vi "NIIE_Classes Initialization.vi"(7 "LabVIEW Icon":string, 8 "Error":errorcluster {"code" min=0 max=0}, 10 "User Events":T8, 11 "Ref Cluster":T3) -> (0 "Error Out":errorcluster {"code" min=0 max=0}, 3 "Data Out":T1={"Class"={"Ants"=refnum, "Layer"=refnum, "Templates"=refnum, "Icon"=refnum, "Glyph"=refnum, "Settings"=refnum, "Tools"=refnum}, "Ref"={"Add Layer"=refnum, "Remove Layer"=refnum, "Line Text"=[], "Body Text Spec"=refnum, "DNL_Font"=refnum, "glyph path str"=refnum, "templates path str"=refnum, "Arrow Up"=refnum, "Arrow Down"=refnum, "IE VI Ref"=refnum, "Glyphs tree"=refnum, "Templates tree"=refnum, "Layer Icon Text"=refnum, "Layer Template"=refnum, "Clipboard"=refnum, "BW icon in"=refnum, "Color icon in"=refnum, "Layer Clust"=refnum, "Body Text"=refnum, "DNL_Framework Templates"=refnum, "Search Templates"=refnum, "TextMarker"=refnum, "Tab Control"=refnum, "Search Glyphs"=refnum, "Line Color"=refnum, "DNL_Glyphs []"=refnum, "Fill Color"=refnum, "Tools"=refnum, "Glyphs tree"=refnum, "Icon"=refnum, "Preview"=refnum, "Ants"=refnum, "Terminals"=refnum, "menu reference"=refnum, "LayerNames"=[], "GlyphLoadAnimation"=refnum, "TemplateLoadAnimation"=refnum, "refreshGlyphs"=refnum, "refreshTemplates"=refnum}, "Support"={"AntsRect"={"left"=0, "top"=0, "right"=0, "bottom"=0}, "Mouse Move Coords"={"Horizontal"=0, "Vertical"=0}, "Mouse Down Coords"={"Horizontal"=0, "Vertical"=0}, "Temp Coord"={"Horizontal"=0, "Vertical"=0}, "Action"=enum."Default", "Edge Color"=4914962, "Fill Color"=16860, "Mouse Down?"=FALSE, "Draft Mode?"=FALSE, "Temp Icon"=bytes[3102], "CTRL Pressed"=FALSE, "Move Selection?"=FALSE, "AntsRect Orig"={"left"=0, "top"=0, "right"=0, "bottom"=0}, "Text"="", "TM Set?"=FALSE, "Mouse inside icon?"=FALSE, "Tool (old value)"=0, "Pencil Move Color"=0, "Swap Colors?"=FALSE, "Shift pressed?"=FALSE}})   [LabVIEW 2021]
uses:
  Controls/References Cluster.ctl
  Controls/IE Data.ctl
  Class/Ants/Ants.lvclass
  Class/FakedArray/FakedArray.lvclass
  Class/Icon Library/Glyph.lvclass
  Class/Settings/Settings.lvclass
  Class/Tools/Tools Paint.lvclass
  vi.lib/LabVIEW Icon API/lv_icon/Classes/Icon/Icon.lvclass
  Controls/IE Classes.ctl
  Controls/SupportClass.ctl
  <vilib>/Utility/miscctls.llb/LVPoint32TypeDef.ctl
  Controls/ENUM_SupportClass_Action.ctl
  vi.lib/LabVIEW Icon API/lv_icon/Controls/IEColor.ctl
  Controls/ToMoreSpecific_Faked2DArray.ctl
  Controls/Undo Redo Action.ctl
  Global Variables/NIIE_Global Data.vi
panel:
  in  "Data":T1={"Class"={"Ants"=refnum, "Layer"=refnum, "Templates"=refnum, "Icon"=refnum, "Glyph"=refnum, "Settings"=refnum, "Tools"=refnum}, "Ref"={"Add Layer"=refnum, "Remove Layer"=refnum, "Line Text"=[], "Body Text Spec"=refnum, "DNL_Font"=refnum, "glyph path str"=refnum, "templates path str"=refnum, "Arrow Up"=refnum, "Arrow Down"=refnum, "IE VI Ref"=refnum, "Glyphs tree"=refnum, "Templates tree"=refnum, "Layer Icon Text"=refnum, "Layer Template"=refnum, "Clipboard"=refnum, "BW icon in"=refnum, "Color icon in"=refnum, "Layer Clust"=refnum, "Body Text"=refnum, "DNL_Framework Templates"=refnum, "Search Templates"=refnum, "TextMarker"=refnum, "Tab Control"=refnum, "Search Glyphs"=refnum, "Line Color"=refnum, "DNL_Glyphs []"=refnum, "Fill Color"=refnum, "Tools"=refnum, "Glyphs tree"=refnum, "Icon"=refnum, "Preview"=refnum, "Ants"=refnum, "Terminals"=refnum, "menu reference"=refnum, "LayerNames"=[], "GlyphLoadAnimation"=refnum, "TemplateLoadAnimation"=refnum, "refreshGlyphs"=refnum, "refreshTemplates"=refnum}, "Support"={"AntsRect"={"left"=0, "top"=0, "right"=0, "bottom"=0}, "Mouse Move Coords"={"Horizontal"=0, "Vertical"=0}, "Mouse Down Coords"={"Horizontal"=0, "Vertical"=0}, "Temp Coord"={"Horizontal"=0, "Vertical"=0}, "Action"=enum."Default", "Edge Color"=4914962, "Fill Color"=16860, "Mouse Down?"=FALSE, "Draft Mode?"=FALSE, "Temp Icon"=bytes[3102], "CTRL Pressed"=FALSE, "Move Selection?"=FALSE, "AntsRect Orig"={"left"=0, "top"=0, "right"=0, "bottom"=0}, "Text"="", "TM Set?"=FALSE, "Mouse inside icon?"=FALSE, "Tool (old value)"=0, "Pencil Move Color"=0, "Swap Colors?"=FALSE, "Shift pressed?"=FALSE}}
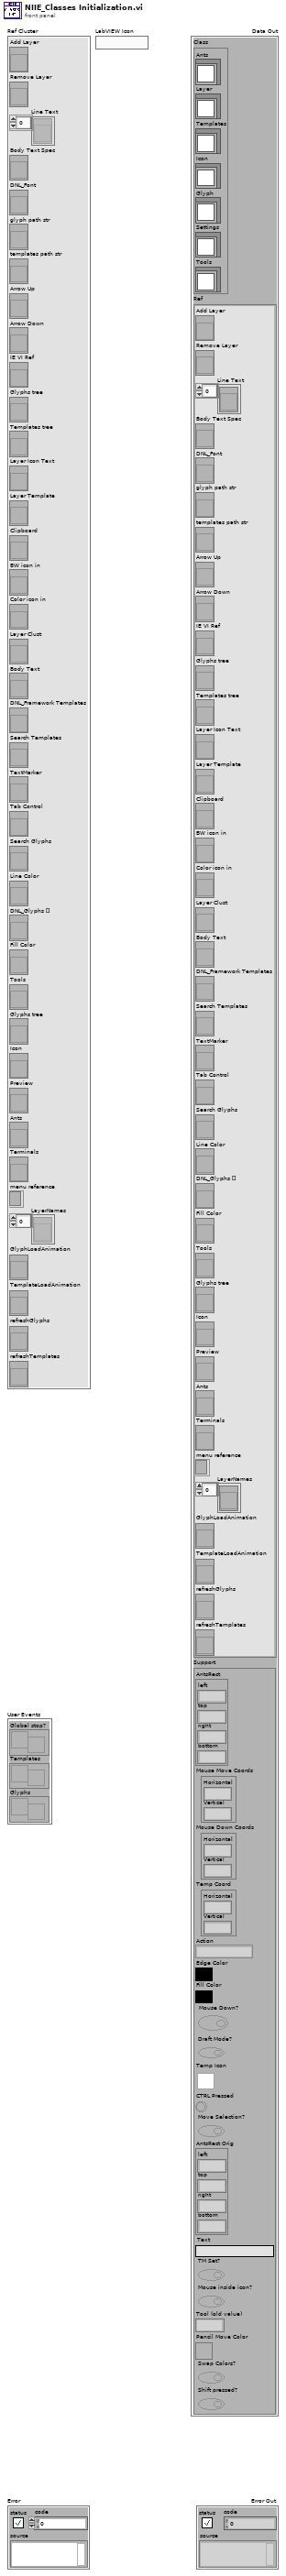
[diagram p1: front panel]
types:
  T1 = typedef "IE Data.ctl" = cluster{"Class":T2, "Ref":T3, "Support":T4}
  T2 = typedef "IE Classes.ctl" = cluster{"Ants":refnum<class "Ants.lvclass">, "Layer":refnum<class "FakedArray.lvclass">, "Templates":refnum<class "FakedArray.lvclass">, "Icon":refnum<class "Icon.lvclass">, "Glyph":refnum<class "Glyph.lvclass">, "Settings":refnum<class "Settings.lvclass">, "Tools":refnum<class "Tools Paint.lvclass">}
  T3 = typedef "References Cluster.ctl" = cluster{"Add Layer":refnum<vi>, "Remove Layer":refnum<vi>, "Line Text":refnum<vi>[], "Body Text Spec":refnum<vi>, "DNL_Font":refnum<vi>, "glyph path str":refnum<vi>, "templates path str":refnum<vi>, "Arrow Up":refnum<vi>, "Arrow Down":refnum<vi>, "IE VI Ref":refnum<vi>, "Glyphs tree":refnum<vi>, "Templates tree":refnum<vi>, "Layer Icon Text":refnum<vi>, "Layer Template":refnum<vi>, "Clipboard":refnum<vi>, "BW icon in":refnum<vi>, "Color icon in":refnum<vi>, "Layer Clust":refnum<vi>, "Body Text":refnum<vi>, "DNL_Framework Templates":refnum<vi>, "Search Templates":refnum<vi>, "TextMarker":refnum<vi>, "Tab Control":refnum<vi>, "Search Glyphs":refnum<vi>, "Line Color":refnum<vi>, "DNL_Glyphs []":refnum<vi>, "Fill Color":refnum<vi>, "Tools":refnum<vi>, "Glyphs tree":refnum<vi>, "Icon":refnum<vi>, "Preview":refnum<vi>, "Ants":refnum<vi>, "Terminals":refnum<vi>, "menu reference":refnum<k9>, "LayerNames":refnum<vi>[], "GlyphLoadAnimation":refnum<vi>, "TemplateLoadAnimation":refnum<vi>, "refreshGlyphs":refnum<vi>, "refreshTemplates":refnum<vi>}
  T4 = typedef "SupportClass.ctl" = cluster{"AntsRect":cluster{"left":i16, "top":i16, "right":i16, "bottom":i16}, "Mouse Move Coords":T5, "Mouse Down Coords":T5, "Temp Coord":T5, "Action":T6, "Edge Color":T7, "Fill Color":T7, "Mouse Down?":bool, "Draft Mode?":bool, "Temp Icon":picture, "CTRL Pressed":bool, "Move Selection?":bool, "AntsRect Orig":cluster{"left":i16, "top":i16, "right":i16, "bottom":i16}, "Text":string, "TM Set?":bool, "Mouse inside icon?":bool, "Tool (old value)":u32, "Pencil Move Color":u32, "Swap Colors?":bool, "Shift pressed?":bool}
  T5 = typedef "LVPoint32TypeDef.ctl" = cluster{"Horizontal":i32, "Vertical":i32}
  T6 = typedef "ENUM_SupportClass_Action.ctl" = enum16{"Default", "Move Selection", "Glyph Library", "Tool"}
  T7 = typedef "IEColor.ctl" = u32
  T8 = cluster{"Global stop?":refnum<user-event>, "Templates":refnum<user-event>, "Glyphs":refnum<user-event>}
  T9 = typedef "Undo Redo Action.ctl" = enum16{"Init", "Add", "Redo", "Undo", "Undo Preview"}
  T10 = typedef "ToMoreSpecific_Faked2DArray.ctl" = enum16{"Framework Templates", "Layer List"}
  T11 = cluster{"Minimum # of selected elements":u32, "Maximum # of selected elements":u32, "# Rows":u32, "# Cols":u32}
  T12 = cluster{"LayerIcon":picture, "LayerName":string, "Opacity":u8, "Visibility?":bool}
  T13 = typedef "Cluster_Layer Data.ctl" = cluster{"LayerIcon":picture, "LayerName":string, "Opacity":u8, "Visibility?":bool}
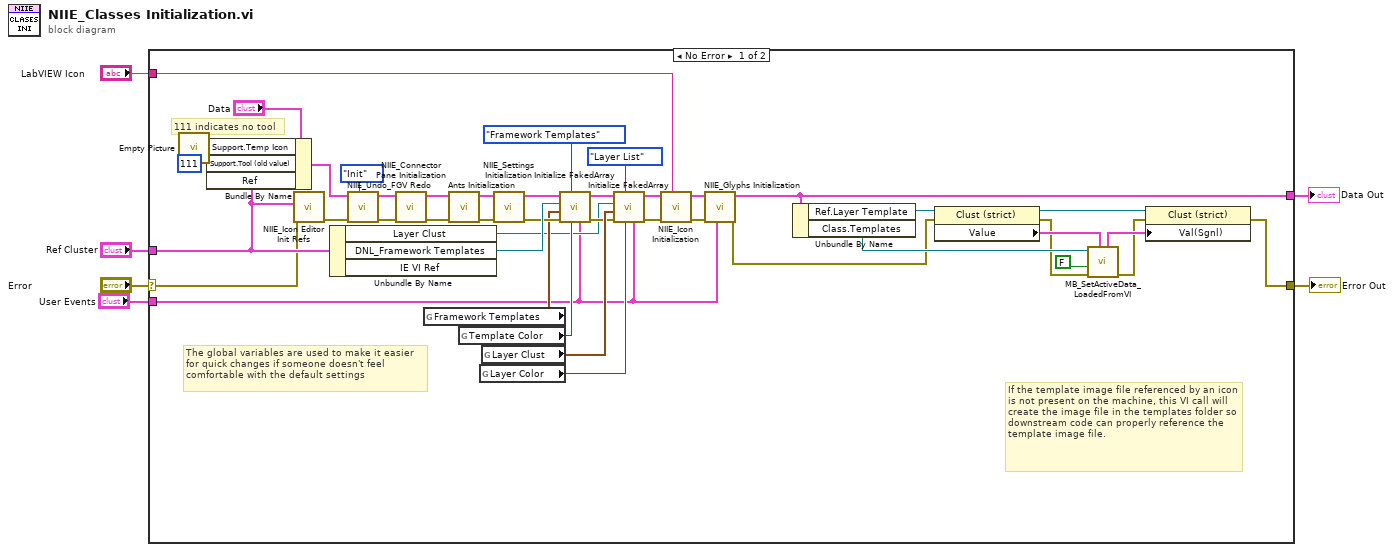
[diagram p0: block diagram]
diagram:
  n1 = case shown="No Error" "Error" {
    selector: "Error" -> [w30 w50]
    tunnel: [w9 w50] -> w5
    tunnel: "Ref Cluster" -> [w35 _]
    tunnel: "User Events" -> [w37 _]
    tunnel: [w17 _] -> w2
    tunnel: "LabVIEW Icon" -> [w18 _]
    frame No Error {
      # "If the template image file referenced by an icon is not present on the machine, this VI call will create the image file in the templates folder so downstream code can properly reference the template image file."
      # "The global variables are used to make it easier\nfor quick changes if someone doesn't feel\ncomfortable with the default settings"
      # "111 indicates no tool"
      n2 = call "Empty Picture"() -> ("empty picture"=w26:picture)
      n3 = Bundle By Name(cluster="Data", "Support.Temp Icon"=w26, "Support.Tool (old value)"=u32 111, "Ref"=w35) -> (w19:T1)
      n4 = call "NIIE_Icon Editor Init Refs.vi"("error in (no error)"=w30, "Ref Cluster"=w35) -> ("error out"=w20:errorcluster)  [unwired: 1 in, 8 out]
      n5 = Unbundle By Name(w35) -> ("Layer Clust"=w40:refnum<vi>, "DNL_Framework Templates"=w49:refnum<vi>)  [unwired: 1 out]
      n6 = call "NIIE_Undo_FGV Redo.vi"("Action"=Undo_Redo_Action."Init", "Error"=w20, "Data"=w19) -> ("Error Out"=w21:errorcluster, "Data Out"=w22:T1)  [unwired: 1 in, 6 out]
      n7 = call "NIIE_Connector Pane Initialization.vi"("Error"=w21, "Data"=w22) -> ("Error Out"=w38:errorcluster, "Data Out"=w31:T1)  [unwired: 8 out]
      n8 = global read "NIIE_Global Data.vi" "Framework Templates"() -> (w45:T11)
      n9 = call "Ants Initialization.vi"("error in (no error)"=w38, "Data in"=w31) -> ("error out"=w39:errorcluster, "Data out"=w34:T1)  [unwired: 8 out]
      n10 = global read "NIIE_Global Data.vi" "Template Color"() -> (w44:T7)
      n11 = global read "NIIE_Global Data.vi" "Layer Color"() -> (w42:T7)
      n12 = global read "NIIE_Global Data.vi" "Layer Clust"() -> (w43:T11)
      n13 = call "NIIE_Settings Initialization.vi"("Error"=w39, "Data"=w34) -> ("Error Out"=w47:errorcluster, "Data Out"=w33:T1)  [unwired: 8 out]
      n14 = call "Initialize FakedArray.vi"("User Events"=w37, "Color"=w44, "ToMoreSpecific"=ToMoreSpecific_Faked2DArray."Framework Templates", "Error"=w47, 9:"Data"=w45, "Cluster Refnum"=w49, 11:"Data"=w33) -> ("Error Out"=w41:errorcluster, "Data Out"=w32:T1)  [unwired: 1 in, 2 out]
      n15 = call "Initialize FakedArray.vi"("User Events"=w37, "Color"=w42, "ToMoreSpecific"=ToMoreSpecific_Faked2DArray."Layer List", "Error"=w41, 9:"Data"=w43, "Cluster Refnum"=w40, 11:"Data"=w32) -> ("Error Out"=w28:errorcluster, "Data Out"=w27:T1)  [unwired: 1 in, 2 out]
      n16 = call "NIIE_Icon Initialization.vi"("LabVIEW Icon"=w18, "Error"=w28, "Data"=w27) -> ("Error Out"=w25:errorcluster, "Data Out"=w24:T1)  [unwired: 7 out]
      n17 = call "NIIE_Glyphs Initialization.vi"("User Events"=w37, "Error"=w25, "Data"=w24) -> ("Error Out"=w8:errorcluster, "Data Out"=w17:T1)  [unwired: 7 out]
      n18 = Unbundle By Name(w17) -> ("Ref.Layer Template"=w14:refnum<vi>, "Class.Templates"=w16:refnum<class "FakedArray.lvclass">)
      n19 = property class="Clust (strict)"(reference=w14, error in=w8) -> (reference out=w12:refnum<vi>, error out=w7:errorcluster, "Value"=w13:T12)
      n20 = call "MB_SetActiveData_LoadedFromVI.vi"("Layer Data"=w13, "Error"=w7, "Match?"=FALSE, "FakedArray"=w16) -> ("Error Out"=w10:errorcluster, "Layer Data Out"=w11:T13)  [unwired: 4 in, 2 out]
      n21 = property class="Clust (strict)"(reference=w12, error in=w10, "Val(Sgnl)"=w11) -> (error out=w9:errorcluster)  [unwired: 1 out]
    }
    frame Error {
    }
  }
  "Error Out" <- w5
  "Data Out" <- w2
